vi "BuildMenu.vi"(8 "error in (no error)":errorcluster, 11 "Menu in":refnum<class "MGI_Menu.lvclass">) -> (0 "error out":errorcluster, 3 "Menu out":refnum<class "MGI_Menu.lvclass">)   [LabVIEW 2016, in "MGI_Menu.lvclass"]
doc: "Iterates through all of the menu (and sub menus) and adds them to the menu.\n\nAuthored by Derek E. Trepanier\nsupport@mooregoodideas.com\nwww.mooregoodideas.com\n\nCopyright (c) 2012, Moore Good Ideas, Inc.\n\nAll rights reserved.\n\nRedistribution and use in source and binary forms, with or without modification, are permitted provided that the following conditions are met:\n\n * Redistributions of source code must retain the above copyright notice, this list of conditions and the following disclaimer.\n * Redistributions in binary form must reproduce the above copyright notice, this list of conditions and the following disclaimer in the documentation and/or other materials provided with the distribution.\n * Neither the name of Moore Good Ideas, Inc. nor the names of its contributors may be used to endorse or promote products derived from this software without specific prior written permission.\n\nTHIS SOFTWARE IS PROVIDED BY THE COPYRIGHT HOLDERS AND CONTRIBUTORS \"AS IS\" AND ANY EXPRESS OR IMPLIED WARRANTIES, INCLUDING, BUT NOT LIMITED TO, THE IMPLIED WARRANTIES OF MERCHANTABILITY AND FITNESS FOR A PARTICULAR PURPOSE ARE DISCLAIMED. IN NO EVENT SHALL THE COPYRIGHT OWNER OR CONTRIBUTORS BE LIABLE FOR ANY DIRECT, INDIRECT, INCIDENTAL, SPECIAL, EXEMPLARY, OR CONSEQUENTIAL DAMAGES (INCLUDING, BUT NOT LIMITED TO, PROCUREMENT OF SUBSTITUTE GOODS OR SERVICES; LOSS OF USE, DATA, OR PROFITS; OR BUSINESS INTERRUPTION) HOWEVER CAUSED AND ON ANY THEORY OF LIABILITY, WHETHER IN CONTRACT, STRICT LIABILITY, OR TORT (INCLUDING NEGLIGENCE OR OTHERWISE) ARISING IN ANY WAY OUT OF THE USE OF THIS SOFTWARE, EVEN IF ADVISED OF THE POSSIBILITY OF SUCH DAMAGE."
uses:
  <userlib>/_MGI/Menu Building/MenuTypes/MGI_Menu.lvclass
  <userlib>/_MGI/Menu Building/MenuTypes/MGI_Menu.lvclass/MGI_Menu.ctl
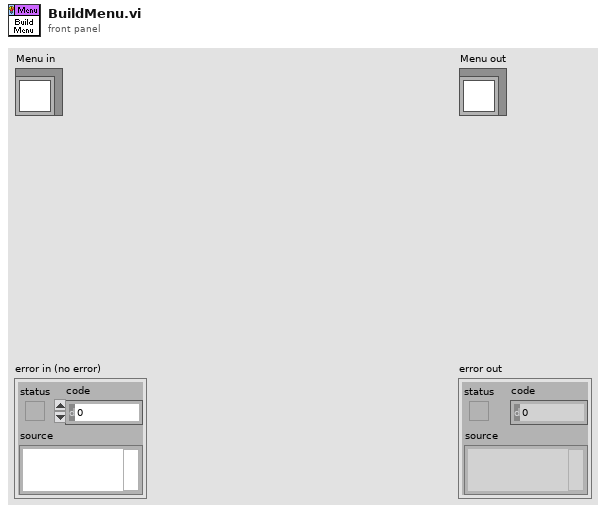
[diagram p1: front panel]
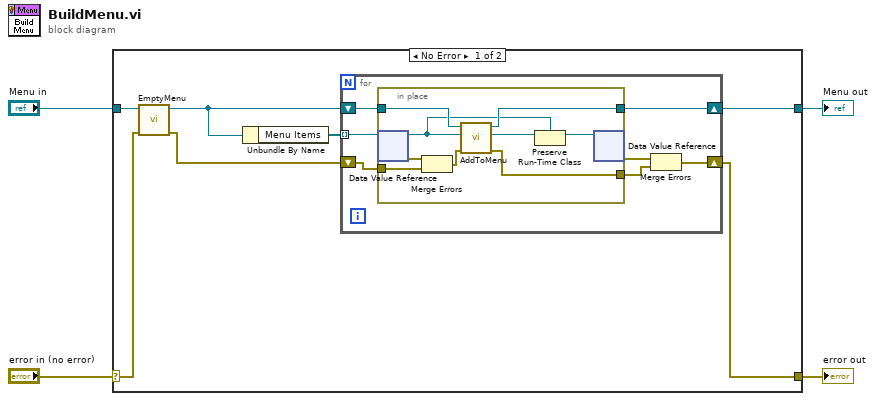
[diagram p0: block diagram]
diagram:
  n1 = case shown="No Error" "error in (no error)" {
    selector: "error in (no error)" -> [w9 w29]
    tunnel: [w8 w29] -> w3
    tunnel: [w5 w28] -> w1
    tunnel: "Menu in" -> [w10 w28]
    frame No Error {
      n2 = call-dynamic "EmptyMenu.vi"("error in (no error)"=w9, "Menu in"=w10) -> ("error out"=w7:errorcluster, "Menu out"=w6:refnum<class "MGI_Menu.lvclass">)  [unwired: 8 in]
      n3 = Unbundle By Name(w6) -> ("Menu Items"=w11:refnum<data-value>[])
      n4 = for {
        tunnel: w11 -> [w16] mode=indexing
        shift-right: [w14] -> w8
        shift-left: w7 -> [w15]
        shift-right: [w12] -> w5
        shift-left: w6 -> [w18]
        n5 = in-place {
          in-place-border: w18 -> [w23]
          in-place-border: [w27] -> w17
          in-place-border: w15 -> [w24]
          in-place-border: [w21] -> w12
          n6 = in-place-dvr #1(w16) -> (w19:refnum<class "MGI_MenuItem.lvclass">, w26:errorcluster)
          n7 = Merge Errors(w26, w24) -> (w25:errorcluster)
          n8 = call-dynamic "AddToMenu.vi"("error in (no error)"=w25, "MenuItem in"=w19, "MGI_Menu in"=w23) -> ("error out"=w27:errorcluster, "MenuItem out"=w22:refnum<class "MGI_MenuItem.lvclass">, "MGI_Menu out"=w21:refnum<class "MGI_Menu.lvclass">)  [unwired: 6 in]
          n9 = Preserve Run-Time Class(object in=w22, 2:w19) -> (object out=w20:refnum<class "MGI_MenuItem.lvclass">)  [unwired: 1 in, 1 out]
          n10 = in-place-dvr #1(w20) -> (w13:errorcluster)  [unwired: 1 out]
        }
        n11 = Merge Errors(w13, w17) -> (w14:errorcluster)
      }
    }
    frame Error {
    }
  }
  "error out" <- w3
  "Menu out" <- w1
